vi "QD Alarm Status.vi"(7 "Set/Check? (F:Set)":bool, 8 "error in (no error)":errorcluster, 9 "Check Parameter (0:Condition)":T1(ring), 10 "Enable Value (0)":u16, 11 "VISA Resource Name":refnum<visa-resource-name>) -> (0 "error out":errorcluster, 1 "Alarm Queue":string[](array[string]), 2 "Bits Set":bool[](array[boolean]), 3 "VISA Resource Name Out":refnum<visa-resource-name>)   [LabVIEW 2012, in "Agilent 34970.lvlib"]
doc: "This VI allows you to set or check the Questionable Data Alarm registers."
uses:
  <instrlib>/Agilent 34970/Agilent 34970.lvlib
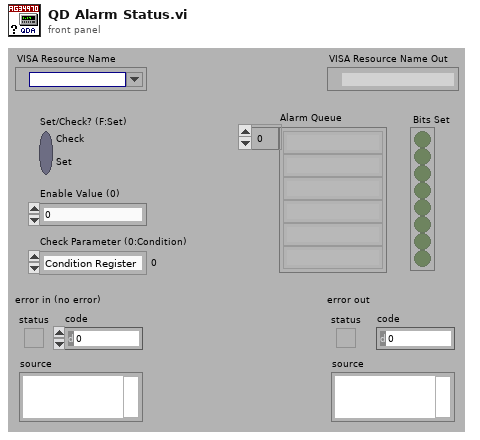
[diagram p1: front panel]
types:
  T1 = enum16{"Condition Register", "Enable Register", "Event Register", "Alarm Queue"}
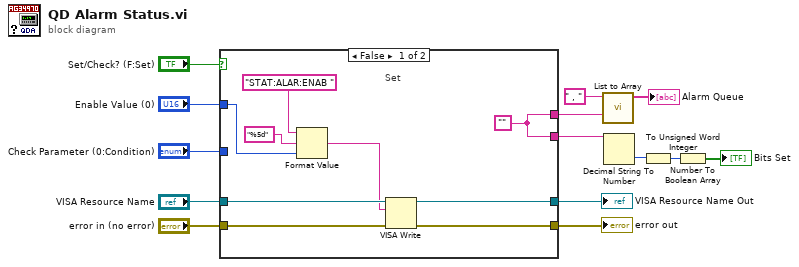
[diagram p0: block diagram]
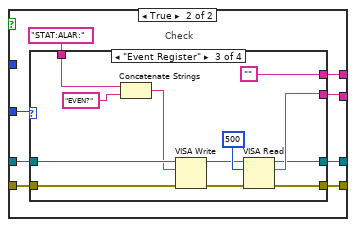
[diagram p2: hidden frame]
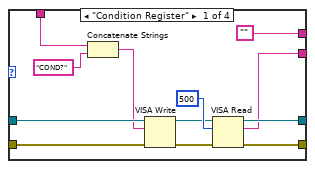
[diagram p3: hidden frame]
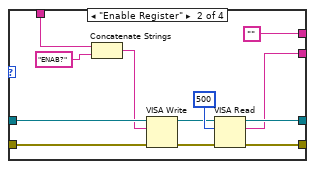
[diagram p4: hidden frame]
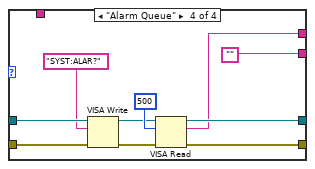
[diagram p5: hidden frame]
diagram:
  n1 = case shown="False" "Set/Check? (F:Set)" {
    tunnel: "Enable Value (0)" -> [w22 _]
    tunnel: "VISA Resource Name" -> [w21 w28]
    tunnel: "error in (no error)" -> [w20 w29]
    tunnel: [w19 w27] -> w3
    tunnel: [w18 w26] -> w5
    tunnel: "Check Parameter (0:Condition)" -> [_ w31]
    tunnel: [w17 w25] -> w11
    tunnel: [w17 w24] -> w8
    frame False {
      w17 = ""
      # "Set"
      n2 = Format Value(string ("")="STAT:ALAR:ENAB ", format string="%5d", value (0)=w22) -> (output string=w15:string)
      n3 = VISA Write(VISA resource name=w21, write buffer=w15, error in (no error)=w20) -> (VISA resource name out=w19:refnum<visa-resource-name>, error out=w18:errorcluster)  [unwired: 1 out]
    }
    frame True {
      # "Check"
      n4 = case shown="\"Event Register\"" w31 {
        tunnel: "STAT:ALAR:" -> [w39 w54 w61 _]
        tunnel: w29 -> [w37 w52 w62 w74]
        tunnel: w28 -> [w38 w51 w63 w71]
        tunnel: [w35 w48 w59 w72] -> w27
        tunnel: [w36 w47 w58 w73] -> w26
        tunnel: [w34 w46 w60 ""] -> w25
        tunnel: ["" "" "" w70] -> w24
        frame "Condition Register" {
          n5 = Concatenate Strings(w39, "COND?" ("multi-line string")) -> (w32:string)
          n6 = VISA Write(VISA resource name=w38, write buffer=w32, error in (no error)=w37) -> (VISA resource name out=w41:refnum<visa-resource-name>, error out=w40:errorcluster)  [unwired: 1 out]
          n7 = VISA Read(VISA resource name=w41, byte count=u32 500 ("byte count (0)"), error in (no error)=w40) -> (VISA resource name out=w35:refnum<visa-resource-name>, read buffer=w34:string, error out=w36:errorcluster)  [unwired: 1 out]
        }
        frame "Enable Register" {
          n8 = Concatenate Strings(w54, "ENAB?" ("multi-line string")) -> (w44:string)
          n9 = VISA Write(VISA resource name=w51, write buffer=w44, error in (no error)=w52) -> (VISA resource name out=w50:refnum<visa-resource-name>, error out=w49:errorcluster)  [unwired: 1 out]
          n10 = VISA Read(VISA resource name=w50, byte count=u32 500 ("byte count (0)"), error in (no error)=w49) -> (VISA resource name out=w48:refnum<visa-resource-name>, read buffer=w46:string, error out=w47:errorcluster)  [unwired: 1 out]
        }
        frame "Event Register" {
          n11 = Concatenate Strings(w61, "EVEN?" ("multi-line string")) -> (w56:string)
          n12 = VISA Write(VISA resource name=w63, write buffer=w56, error in (no error)=w62) -> (VISA resource name out=w65:refnum<visa-resource-name>, error out=w64:errorcluster)  [unwired: 1 out]
          n13 = VISA Read(VISA resource name=w65, byte count=u32 500 ("byte count (0)"), error in (no error)=w64) -> (VISA resource name out=w59:refnum<visa-resource-name>, read buffer=w60:string, error out=w58:errorcluster)  [unwired: 1 out]
        }
        frame "Alarm Queue" {
          n14 = VISA Write(VISA resource name=w71, write buffer="SYST:ALAR?", error in (no error)=w74) -> (VISA resource name out=w76:refnum<visa-resource-name>, error out=w75:errorcluster)  [unwired: 1 out]
          n15 = VISA Read(VISA resource name=w76, byte count=u32 500 ("byte count (0)"), error in (no error)=w75) -> (VISA resource name out=w72:refnum<visa-resource-name>, read buffer=w70:string, error out=w73:errorcluster)  [unwired: 1 out]
        }
      }
    }
  }
  "error out" <- w5
  "VISA Resource Name Out" <- w3
  n16 = call <instrlib>:"List to Array.vi"("List (empty)"=w8, "Separator (,)"=" , " ("Separator")) -> ("Output String Array"=→"Alarm Queue":string[])  [unwired: 8 in, 1 out]
  n17 = Decimal String To Number(string=w11) -> (number=w10:i32)  [unwired: 2 in, 1 out]
  n18 = To Unsigned Word Integer(number=w10) -> (unsigned 16bit integer=w9:u16)
  n19 = Number To Boolean Array(number=w9) -> (Boolean array=→"Bits Set":bool[])
